vi "XY图Y轴范围调整.vi"(6 "留白比例":cluster{"顶白比例":dbl, "底白比例":dbl}={"顶白比例"=0.1, "底白比例"=0.1}, 7 "最值":cluster{"Y-max":dbl, "Y-min":dbl}, 10 "下限模式":enum16{"自由下限", "下限为0"}(ring), 11 "XY图引用":refnum<vi>) -> (1 "Y轴全长":dbl, 2 "新Y标尺.范围":T1 caption="Y标尺.范围", 3 "XY图引用输出":refnum<vi>)   [LabVIEW 2017]
uses:
  <vilib>/Utility/miscctls.llb/LVRangeTypeDef.ctl
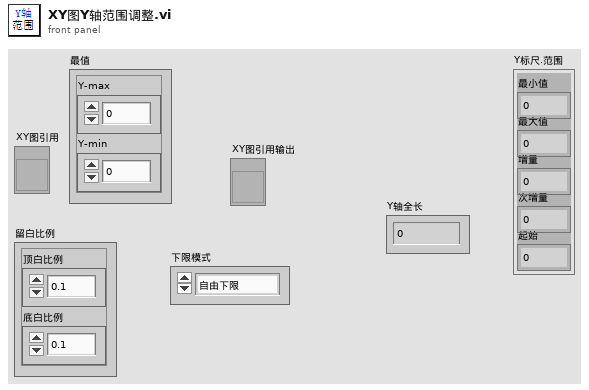
[diagram p1: front panel]
types:
  T1 = typedef "LVRangeTypeDef.ctl" = cluster{"Minimum":dbl, "Maximum":dbl, "Increment":dbl, "Minor Increment":dbl, "Start":dbl}
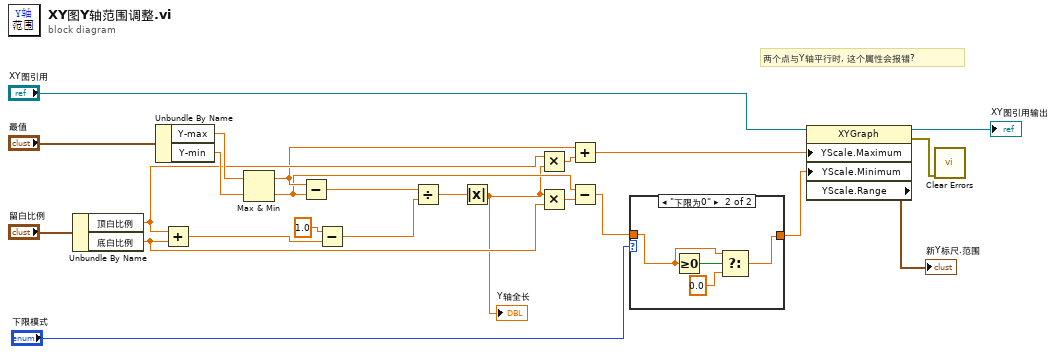
[diagram p0: block diagram]
diagram:
  # "两个点与Y轴平行时, 这个属性会报错?"
  n1 = Unbundle By Name("留白比例") -> ("顶白比例"=w15:dbl, "底白比例"=w13:dbl)
  n2 = Unbundle By Name("最值") -> ("Y-max"=w21:dbl, "Y-min"=w20:dbl)
  n3 = Add(x=w15, y=w13) -> (x+y=w18:dbl)
  n4 = Max & Min(x=w21, y=w20) -> (max(x,y)=w11:dbl, min(x,y)=w10:dbl)
  n5 = Subtract(x=w11, y=w10) -> (x-y=w17:dbl)
  n6 = Subtract(x=1.0, y=w18) -> (x-y=w16:dbl)
  n7 = Divide(x=w17, y=w16) -> (x/y=w14:dbl)
  n8 = Absolute Value(x=w14) -> (abs(x)=w5:dbl)
  "Y轴全长" <- w5
  n9 = Multiply(x=w15, y=w5) -> (x*y=w12:dbl)
  n10 = Multiply(x=w5, y=w13) -> (x*y=w9:dbl)
  n11 = Add(x=w11, y=w12) -> (x+y=w8:dbl)
  n12 = Subtract(x=w10, y=w9) -> (x-y=w3:dbl)
  n13 = case shown="\"下限为0\"" "下限模式" {
    tunnel: w3 -> [w25 w28]
    tunnel: [w25 w26] -> w2
    frame "自由下限", Default {
    }
    frame "下限为0" {
      n14 = Greater Or Equal To 0?(x=w28) -> (x >= 0?=w29:bool)
      n15 = Select(t=w28, s=w29, f=0.0) -> (s? t:f=w26:dbl)
    }
  }
  n16 = property class="XYGraph"(reference="XY图引用", "YScale.Maximum"=w8, "YScale.Minimum"=w2) -> (reference out=→"XY图引用输出":refnum<vi>, error out=w1:errorcluster, "YScale.Range"=→"新Y标尺.范围":T1)  [unwired: 1 in]
  n17 = call <vilib>:"Clear Errors.vi"("error in (no error)"=w1) -> ()  [unwired: 5 in, 2 out]
